vi "generate target 2.vi"(8 "Array":cluster{"Numeric":dbl, "Numeric 2":dbl}[](array[cluster]), 10 "BG Pic":picture) -> (2 "2D Picture":picture)   [LabVIEW 2014]
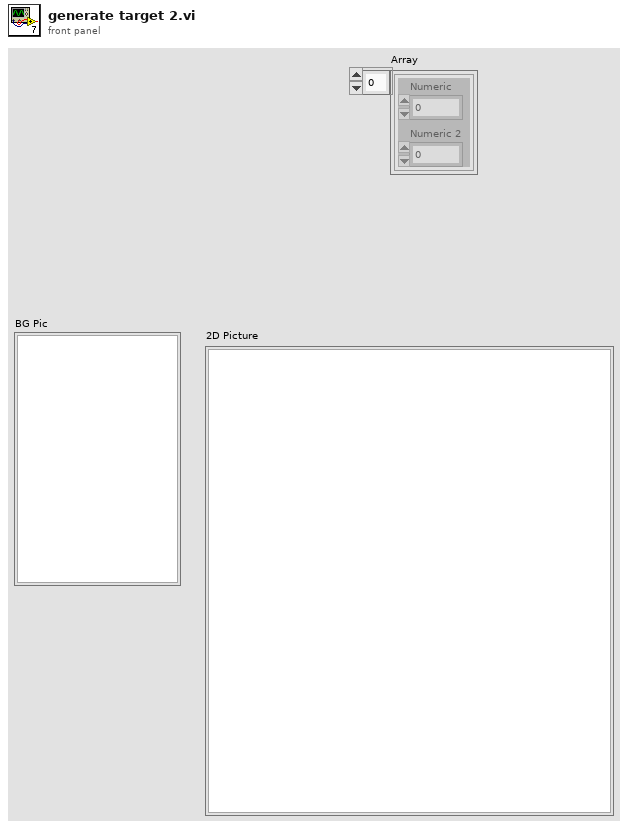
[diagram p1: front panel]
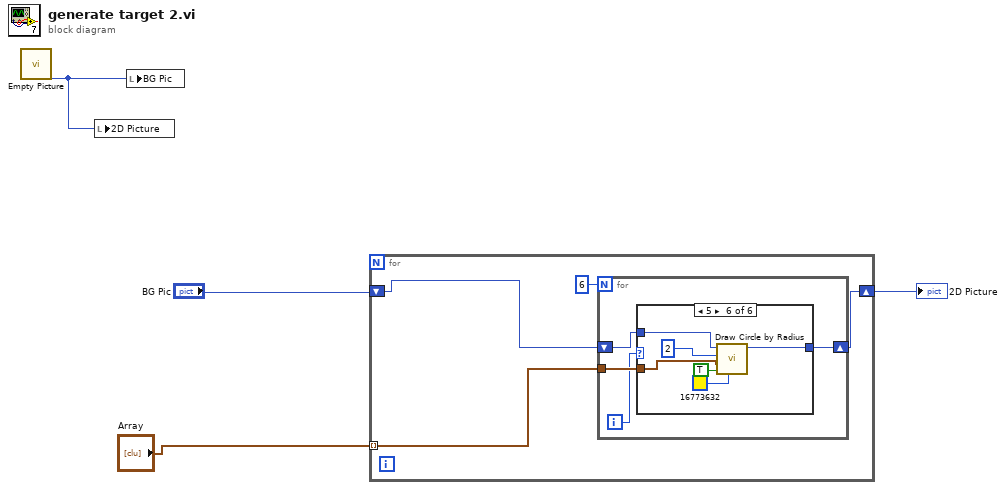
[diagram p0: block diagram]
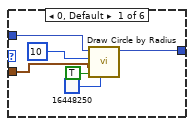
[diagram p2: hidden frame]
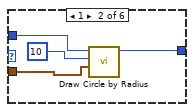
[diagram p3: hidden frame]
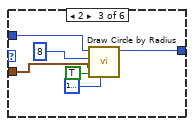
[diagram p4: hidden frame]
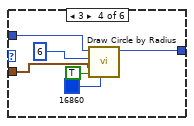
[diagram p5: hidden frame]
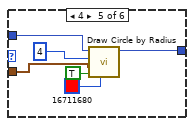
[diagram p6: hidden frame]
diagram:
  n1 = call "Empty Picture"() -> ("empty picture"=w2:picture)
  n2 = local write "2D Picture"(w2) -> ()
  n3 = local write "BG Pic"(w2) -> ()
  n4 = for {
    shift-right: [w8] -> w4
    shift-left: "BG Pic" -> [w6]
    tunnel: "Array" -> [w5] mode=indexing
    n5 = for {
      N: 6 -> [_]
      tunnel: w5 -> [w12]
      shift-right: [w11] -> w8
      shift-left: w6 -> [w9]
      i -> [w10]
      n6 = case shown="5" w10 {
        tunnel: w12 -> [w18 w22 w28 w34 w40 w46]
        tunnel: [w17 w21 w27 w33 w39 w45] -> w11
        tunnel: w9 -> [w13 w19 w23 w29 w35 w41]
        frame 0, Default {
          n7 = call <vilib>:"Draw Circle by Radius.vi"("color(black)"=u32 16448250, "fill?(F)"=TRUE, "pixel center"=w18, "radius"=i16 10, "picture"=w13) -> ("new picture"=w17:picture)  [unwired: 6 in]
        }
        frame 1 {
          n8 = call <vilib>:"Draw Circle by Radius.vi"("pixel center"=w22, "radius"=i16 10, "picture"=w19) -> ("new picture"=w21:picture)  [unwired: 8 in]
        }
        frame 2 {
          n9 = call <vilib>:"Draw Circle by Radius.vi"("color(black)"=u32 16777222, "fill?(F)"=TRUE, "pixel center"=w28, "radius"=i16 8, "picture"=w23) -> ("new picture"=w27:picture)  [unwired: 6 in]
        }
        frame 3 {
          n10 = call <vilib>:"Draw Circle by Radius.vi"("color(black)"=u32 16860, "fill?(F)"=TRUE, "pixel center"=w34, "radius"=i16 6, "picture"=w29) -> ("new picture"=w33:picture)  [unwired: 6 in]
        }
        frame 4 {
          n11 = call <vilib>:"Draw Circle by Radius.vi"("color(black)"=u32 16711680, "fill?(F)"=TRUE, "pixel center"=w40, "radius"=i16 4, "picture"=w35) -> ("new picture"=w39:picture)  [unwired: 6 in]
        }
        frame 5 {
          n12 = call <vilib>:"Draw Circle by Radius.vi"("color(black)"=u32 16773632, "fill?(F)"=TRUE, "pixel center"=w46, "radius"=i16 2, "picture"=w41) -> ("new picture"=w45:picture)  [unwired: 6 in]
        }
      }
    }
  }
  "2D Picture" <- w4
